vi "EFW Set Position.vi"(8 "error in (no error)":errorcluster caption="错误输入（无错误）", 10 "Position":i32, 11 "ID":i32) -> (0 "error out":errorcluster caption="错误输出", 3 "function return":u32(ring))   [LabVIEW 2012, in "EFW_filter.lvlib"]
doc: "EFW_API EFW_ERROR_CODE EFWSetPosition(int ID, int Position);"
uses:
  <userlib>/EFW_filter/EFW_filter.lvlib
  <userlib>/EFW_filter/EFW_filter.dll
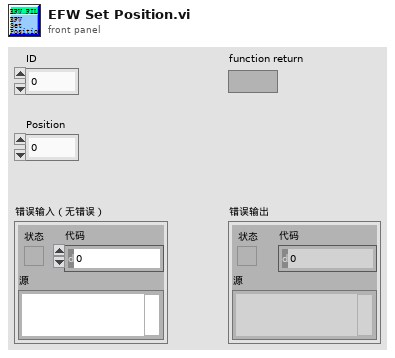
[diagram p1: front panel]
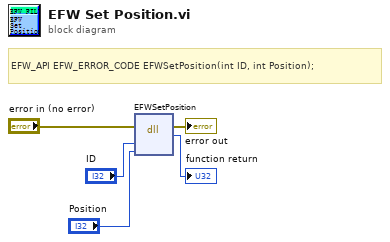
[diagram p0: block diagram]
diagram:
  # "EFW_API\tEFW_ERROR_CODE EFWSetPosition(int ID, int Position);"
  n1 = dll-call lib="D:/Program Files (x86)/National Instruments/LabVIEW 2012/user.lib/EFW_filter/EFW_filter.*" fn="EFWSetPosition"(error in="error in (no error)", "ID"="ID", "Position"="Position") -> (error out=→"error out":errorcluster, →"function return":u32)  [unwired: 4 in, 1 out]
